vi "calAlign.vi"(8 "offset":i32, 9 "Decimated 660":dbl[](array[numeric]), 10 "Decimated 532":dbl[](array[numeric]), 11 "GO3 Data":dbl[](array[numeric])) -> (3 "Aligned Data":cluster{"Array":i32[], "Decimated 660":dbl[]}[](array[cluster]))   [LabVIEW 2011]
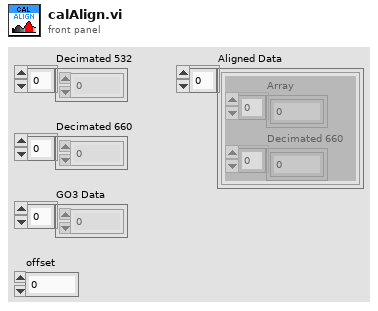
[diagram p1: front panel]
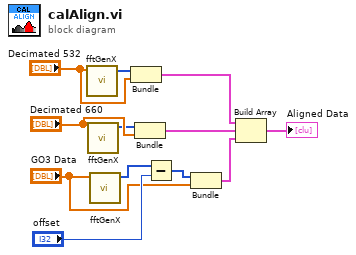
[diagram p0: block diagram]
diagram:
  n1 = call "fftGenX.vi"("Output Array"="Decimated 532") -> ("Array"=w4:i32[])  [unwired: 10 in]
  n2 = call "fftGenX.vi"("Output Array"="Decimated 660") -> ("Array"=w5:i32[])  [unwired: 10 in]
  n3 = call "fftGenX.vi"("Output Array"="GO3 Data") -> ("Array"=w9:i32[])  [unwired: 10 in]
  n4 = Bundle("Array"=w4, "Decimated 532"="Decimated 532") -> (w7:cluster{"Array":i32[], "Decimated 532":dbl[]})  [unwired: 1 in]
  n5 = Bundle("Array"=w5, "Decimated 660"="Decimated 660") -> (w8:cluster{"Array":i32[], "Decimated 660":dbl[]})  [unwired: 1 in]
  n6 = Subtract(x=w9, y="offset") -> (x-y=w10:i32[])
  n7 = Bundle(w10, "GO3 Data"="GO3 Data") -> (w3:cluster{i32[], "GO3 Data":dbl[]})  [unwired: 1 in]
  n8 = Build Array(w7, w8, w3) -> (→"Aligned Data":cluster{"Array":i32[], "GO3 Data":dbl[]}[])
